vi "parmsQSB.vi"(1 "dimensions":i64[](array[numeric])=[1399090569999999999, -1], 2 "values":T1(array[cluster])=[{"Nchannel"=96, "ADCbits"=16, "BridgeVoltage (V)"=5.0, "ExptSampleFrequency (Hz)"=1250.0, "CalSampleFrequency (Hz)"=1250.0, "CalStep1 (V)"="2.5", "CalStep2 (V)"="3.7", "detector"="Au_Kapton"}], 3 "label":string="parms") -> (0 "JSON string":string="{\"label\":\"parms\",\"values\":[{\"Nchannel\":96,\"ADCbits\":16,\"BridgeVoltage (V)\":5,\"ExptSampleFrequency (Hz)\":1250,\"CalSampleFrequency (Hz)\":1250,\"CalStep1 (V)\":\"2.5\",\"CalStep2 (V)\":\"3.7\",\"detector\":\"Au_Kapton\"}],\"dimensions\":[1399090569999999999,-1]}")   [LabVIEW 2014]
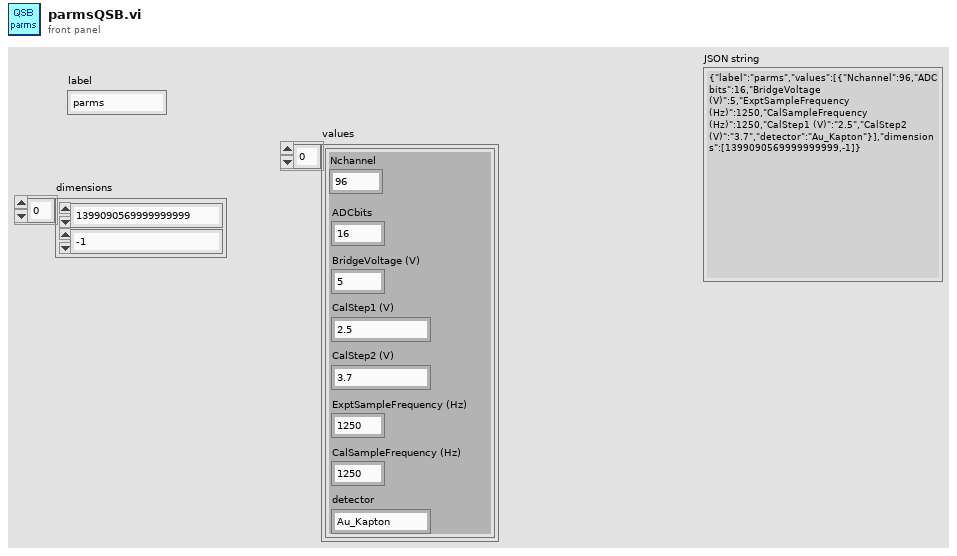
[diagram p1: front panel]
types:
  T1 = cluster{"Nchannel":i16, "ADCbits":i16, "BridgeVoltage (V)":sgl, "ExptSampleFrequency (Hz)":sgl, "CalSampleFrequency (Hz)":sgl, "CalStep1 (V)":string, "CalStep2 (V)":string, "detector":string}[]
  T2 = cluster{"label":string, "values":cluster{"Nchannel":i16, "ADCbits":i16, "BridgeVoltage (V)":sgl, "ExptSampleFrequency (Hz)":sgl, "CalSampleFrequency (Hz)":sgl, "CalStep1 (V)":string, "CalStep2 (V)":string, "detector":string}[], "dimensions":i64[]}
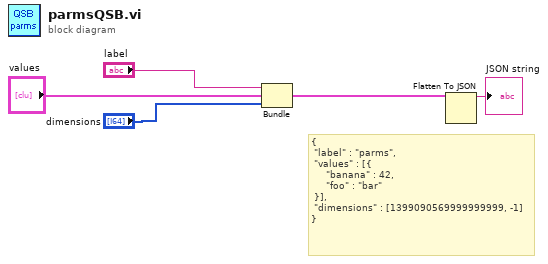
[diagram p0: block diagram]
diagram:
  # "{\n \"label\" : \"parms\",\n \"values\" : [{\n     \"banana\" : 42,\n     \"foo\" : \"bar\"\n }],\n \"dimensions\" : [1399090569999999999, -1]\n}"
  n1 = Bundle("label"="label", "values"="values", "dimensions"="dimensions") -> (w2:T2)  [unwired: 1 in]
  n2 = Flatten To JSON(anything=w2) -> (JSON string=→"JSON string":string)  [unwired: 2 in, 1 out]
